vi "Pipelined Burst FFT Core SGL.vi"(9 "xn_im":fxp<+,32,32>, 10 "xn_re":fxp<+,32,32>, 11 "FFT State Info In":T2) -> (0 "Output Valid":bool, 1 "Output_Imaginary":fxp<+,32,32>, 2 "Output_Real":fxp<+,32,32>, 3 "FFT Output":T1, 4 "FFT Output Index":fxp<+,11,11>, 6 "edone":bool)   [LabVIEW 2012]
doc: "This FFT Core is currently configured to run for 512 points"
uses:
  <vilib>/rvi/IPIntegrationNode/IPINode_Utilities/niFpgaIPINodeSimCore.vi
  <vilib>/rvi/FXPMathLib/basic elements/FxpDiscreteDelay/XNode/nifxpmath_DiscreteDelay.xnode
  <vilib>/rvi/XilinxIP/XIPIN_XNode/niFpgaXIPIN.xnode
  <userlib>/FPGA Library/Code Development/Signal Processing/FFT/Pipelined Burst FFT/Xilinx FFT Core SGL/XilinxFFTCoreSGL_9831F7DF46872FC4236071A27A2EF98C.dll
  <vilib>/rvi/IPIntegrationNode/IPINode_Xnode/niFpgaIPINode.xnode
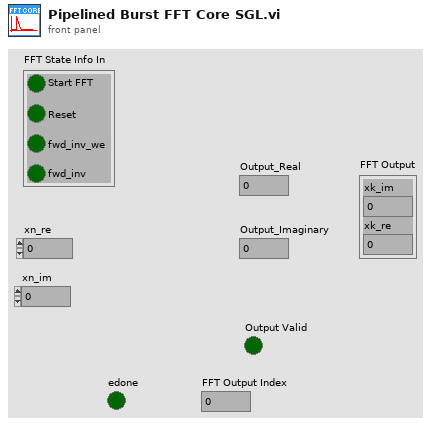
[diagram p1: front panel]
types:
  T1 = cluster{"xk_im":fxp<+,32,32>, "xk_re":fxp<+,32,32>}
  T2 = cluster{"Reset":bool, "Start FFT":bool, "fwd_inv_we":bool, "fwd_inv":bool}
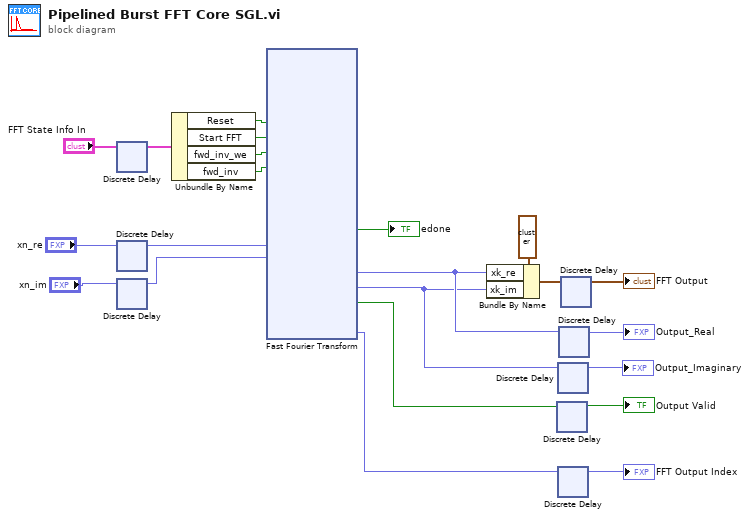
[diagram p0: block diagram]
diagram:
  n1 = xnode "Discrete Delay"("D"="FFT State Info In") -> ("Q"=w11:T2)
  n2 = xnode "Discrete Delay"("D"="xn_re") -> ("Q"=w10:fxp<+,32,32>)
  n3 = xnode "Discrete Delay"("D"="xn_im") -> ("Q"=w9:fxp<+,32,32>)
  n4 = Unbundle By Name(w11) -> ("Reset"=w17:bool, "Start FFT"=w16:bool, "fwd_inv_we"=w15:bool, "fwd_inv"=w14:bool)
  n5 = xnode ("Fast Fourier Transform")("sclr"=w17, "start"=w16, "fwd_inv_we"=w15, "fwd_inv"=w14, "xn_re"=w10, "xn_im"=w9) -> ("edone"=→"edone":bool, "xk_re"=w4:fxp<+,32,32>, "xk_im"=w3:fxp<+,32,32>, "dv"=w20:bool, "xk_index"=w5:fxp<+,11,11>)  [unwired: 4 out]
  n6 = Bundle By Name(cluster=T1 {"xk_im"=0.0, "xk_re"=0.0} ("FFT Output"), "xk_re"=w4, "xk_im"=w3) -> (w12:T1)
  n7 = xnode "Discrete Delay"("D"=w20) -> ("Q"=→"Output Valid":bool)
  n8 = xnode "Discrete Delay"("D"=w3) -> ("Q"=→"Output_Imaginary":fxp<+,32,32>)
  n9 = xnode "Discrete Delay"("D"=w5) -> ("Q"=→"FFT Output Index":fxp<+,11,11>)
  n10 = xnode "Discrete Delay"("D"=w4) -> ("Q"=→"Output_Real":fxp<+,32,32>)
  n11 = xnode "Discrete Delay"("D"=w12) -> ("Q"=→"FFT Output":T1)
